vi "DAQmx_QMH_DO_LED_Switch.vi"() -> ()   [LabVIEW 2015]
uses:
  <vilib>/DAQmx/write.llb/DAQmx Write (Digital Bool 1Line 1Point).vi
  <vilib>/DAQmx/create/channels.llb/DAQmx Create Channel (DO-Digital Output).vi
  <vilib>/DAQmx/miscellaneous.llb/DAQmx Fill In Error Info.vi
panel:
  out "Boolean":bool
  in  "Stop Button":bool
  in  "Switch":bool
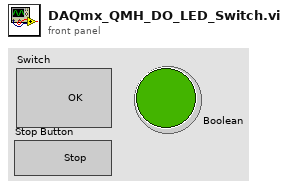
[diagram p1: front panel]
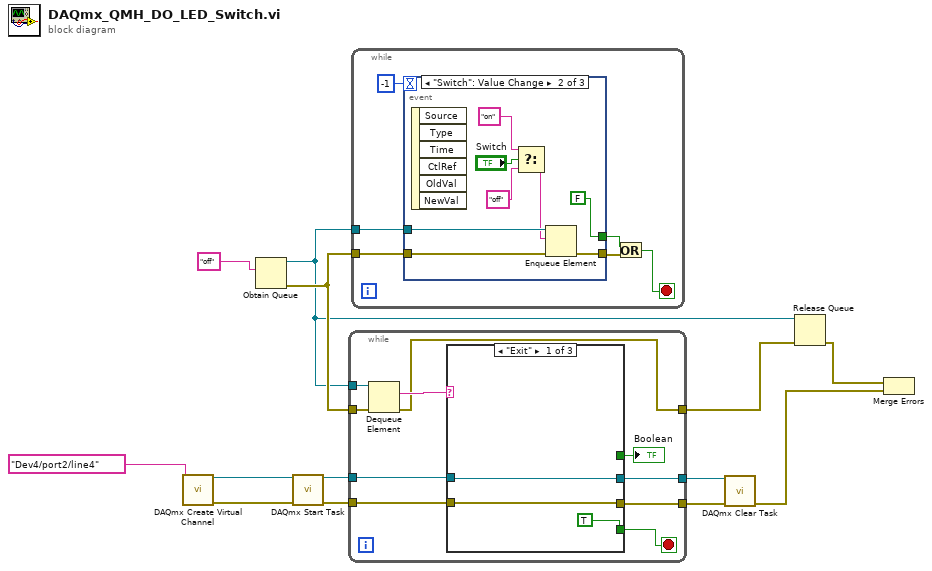
[diagram p0: block diagram]
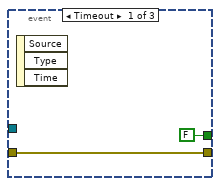
[diagram p2: hidden frame]
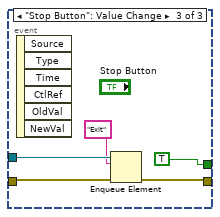
[diagram p3: hidden frame]
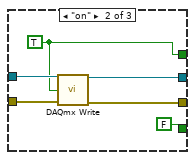
[diagram p4: hidden frame]
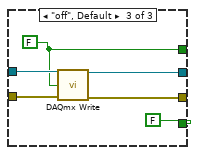
[diagram p5: hidden frame]
diagram:
  n1 = call-poly <vilib>:"DAQmx Create Virtual Channel.vi"("lines"=tag "Dev4/port2/line4") -> ("task out"=w12:refnum<k21>, "error out"=w11:errorcluster)  [unwired: 13 in]
  n2 = Obtain Queue(element data type="off") -> (queue out=w5:refnum<queue>, error out=w6:errorcluster)  [unwired: 4 in, 1 out]
  n3 = call <vilib>:"DAQmx Start Task.vi"("task/channels in"=w12, "error in"=w11) -> ("task out"=w10:refnum<k21>, "error out"=w9:errorcluster)  [unwired: 12 in]
  n4 = while {
    tunnel: w10 -> [w23]
    tunnel: w9 -> [w17]
    tunnel: [w22] -> w8
    tunnel: [w21] -> w7
    tunnel: w5 -> [w20]
    tunnel: w6 -> [w19]
    tunnel: [w16] -> w4
    stop <- w15 stop-if-true
    n5 = Dequeue Element(queue=w20, error in (no error)=w19) -> (element=w18:string, error out=w16:errorcluster)  [unwired: 1 in, 2 out]
    n6 = case shown="\"Exit\"" w18 {
      tunnel: w23 -> [w25 w32 w38]
      tunnel: w17 -> [w24 w31 w37]
      tunnel: [w25 w30 w36] -> w22
      tunnel: [w24 w29 w35] -> w21
      tunnel: [TRUE FALSE FALSE] -> w15
      tunnel: [_ w27 w33] -> w14
      frame "Exit" {
      }
      frame "on" {
        w27 = TRUE
        n7 = call-poly <vilib>:"DAQmx Write.vi"("task/channels in"=w32, "data"=w27, "error in"=w31) -> ("task out"=w30:refnum<k21>, "error out"=w29:errorcluster)  [unwired: 10 in, 1 out]
      }
      frame "off", Default {
        w33 = FALSE ("data")
        n8 = call-poly <vilib>:"DAQmx Write.vi"("task/channels in"=w38, "data"=w33, "error in"=w37) -> ("task out"=w36:refnum<k21>, "error out"=w35:errorcluster)  [unwired: 10 in, 1 out]
      }
    }
    "Boolean" <- w14
  }
  n9 = while {
    tunnel: w5 -> [w43]
    tunnel: w6 -> [w42]
    stop <- w39 stop-if-true
    n10 = event shown="[1] \"Switch\": Value Change" {
      selector: _ -> [_ _ _]
      dyn-events: _ -> [_ _ _]
      timeout: -1 -> [_ _ _]
      tunnel: w43 -> [_ w54 w58]
      tunnel: w42 -> [w46 w53 w59]
      tunnel: [w46 w52 w57] -> w41
      tunnel: [FALSE FALSE TRUE] -> w40
      event Timeout {
        n11 = event-data() -> ()  [unwired: 1 in, 3 out]
      }
      event "Switch": Value Change {
        n12 = event-data() -> ()  [unwired: 1 in, 6 out]
        n13 = Select(t="on", s="Switch", f="off") -> (s? t:f=w50:string)
        n14 = Enqueue Element(queue=w54, element=w50, error in (no error)=w53) -> (error out=w52:errorcluster)  [unwired: 1 in, 2 out]
      }
      event "Stop Button": Value Change {
        n15 = event-data() -> ()  [unwired: 1 in, 6 out]
        n16 = Enqueue Element(queue=w58, element="Exit", error in (no error)=w59) -> (error out=w57:errorcluster)  [unwired: 1 in, 2 out]
      }
    }
    n17 = Or(x=w40, y=w41) -> (x .or. y?=w39:bool)
  }
  n18 = call <vilib>:"DAQmx Clear Task.vi"("task in"=w8, "error in"=w7) -> ("error out"=w2:errorcluster)  [unwired: 13 in]
  n19 = Release Queue(queue=w5, error in (no error)=w4) -> (error out=w3:errorcluster)  [unwired: 1 in, 2 out]
  n20 = Merge Errors(w3, w2) -> ()  [unwired: 1 out]
